vi "AFMss_control_trajTrack.vi"() -> ()   [LabVIEW 2017]
uses:
  controls/controlParams_tracktraj.ctl
  <vilib>/rvi/Emulation/niFpgaGetClockAttributes.vi
  <vilib>/rvi/Emulation/niFpgaSctlEmulationGetInTimedLoop.vi
  <vilib>/rvi/Emulation/niFpgaEmulationReportErrorSimple.vi
  <vilib>/rvi/eio/common/nirviEmuTemplateMethod_errors.vi
  <vilib>/rvi/Emulation/niFpgaCriticalErrorInLSC.vi
  <vilib>/rvi/DataTransferAndStorage/Container/Common/niFpgaContainerExecOnDevCompGetState.vi
  <vilib>/rvi/Emulation/niFpgaEmulationIsFPGAContextNoSignature.vi
  <vilib>/rvi/DataTransferAndStorage/Container/Common/niFpgaContainerGetUniqueNameForEmu.vi
  <vilib>/rvi/Memory/Memory_Emulation/niFpgaMemoryEmulationCacheClearOnFirstRun.vi
  <vilib>/rvi/Memory/Memory_Emulation/nirvimemoryEmulationManagerCache_MakeExclusive.vi
  <vilib>/rvi/Memory/Memory_Emulation/niFpgaMemoryEmulationValidateCache.vi
  <vilib>/rvi/Memory/Memory_Emulation/nirvimemoryEmulationManagerCache_InsertValue.vi
  <vilib>/Utility/error.llb/Clear Errors.vi
  <vilib>/rvi/Memory/Memory_Emulation/nirvimemoryEmulationManagerCache_ReleaseExclusive.vi
  <vilib>/rvi/Memory/Memory_Emulation/nirvimemoryEmulationManagerCache_GetValue.vi
  <vilib>/rvi/Memory/Memory_Emulation/nirvimemoryEmulationManagerCache_SetValue.vi
  <vilib>/rvi/Emulation/niFpgaProcessEmulError.vi
  <vilib>/rvi/interface/RandomDataEmulation/niFpgaRandomDataHandleErrors.vi
  <vilib>/eio/EIONode/EIONode.xnode
  <vilib>/rvi/DataTransferAndStorage/Container/XNode/niFpgaContainer.xnode
  <vilib>/rvi/DataTransferAndStorage/Register/Emulation/niFpgaRegisterEmulationRefIn.vi
  <vilib>/rvi/interface/RandomDataEmulation/nirviRandomDataFpgaReadWriteTemplate.vi
  <vilib>/rvi/FXPMathLib/FxpSub/XNode/nifxpmath_Sub.xnode
  <vilib>/rvi/FXPMathLib/sim/FxpSim.dll
panel:
  out "yk":sgl
  out "u_xk":sgl
  out "yuxk TO":bool
  out "YK TO":bool
  out "UK TO":bool
  in  "Cluster":T1={"umax"=3.0, "y_ref(k)"=0.0, "Ki"=0.0, "y(k) (from plant)"=0.0, "ND"=0, "NS"=0, "u_Kx_ref(k)"=0.0} {"u_Kx_ref(k)" format="%#_13g"; "Ki" format="%#_13g"; "y_ref(k)" format="%#_13g"; "umax" format="%#_13g"}
  out "Unstable Traj":bool
  out "Loop Done":bool
  in  "Settle Ticks":i16=1000
  in  "False  = cont run":bool=TRUE
  in  "Abort":bool=TRUE
  in  "iters":i16=1
  in  "ymax":sgl=4.0 format="%#_13g"
  in  "TsTicks":i16
  out "Loop Ticks (benchmark)":i16
  out "NS":i16=2
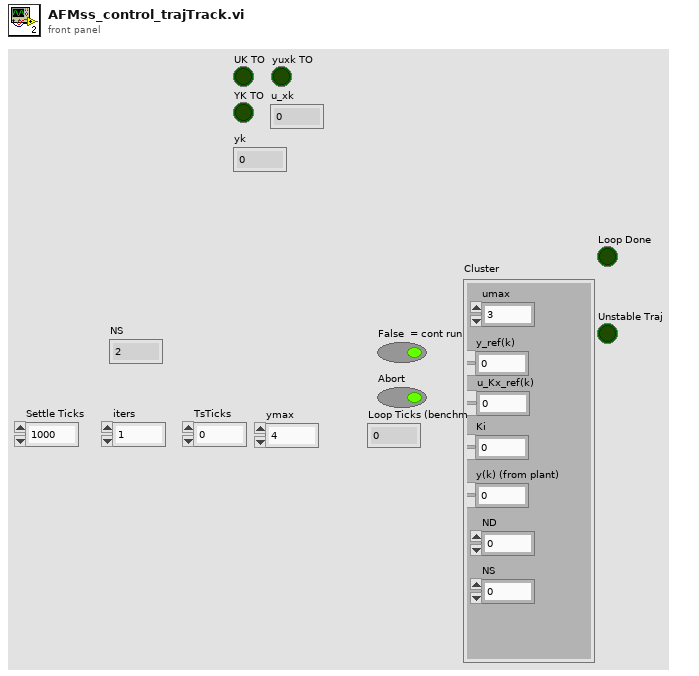
[diagram p1: front panel]
types:
  T1 = typedef "controlParams_tracktraj.ctl" = cluster{"umax":sgl, "y_ref(k)":sgl, "Ki":sgl, "y(k) (from plant)":sgl, "ND":i16, "NS":i16, "u_Kx_ref(k)":sgl}
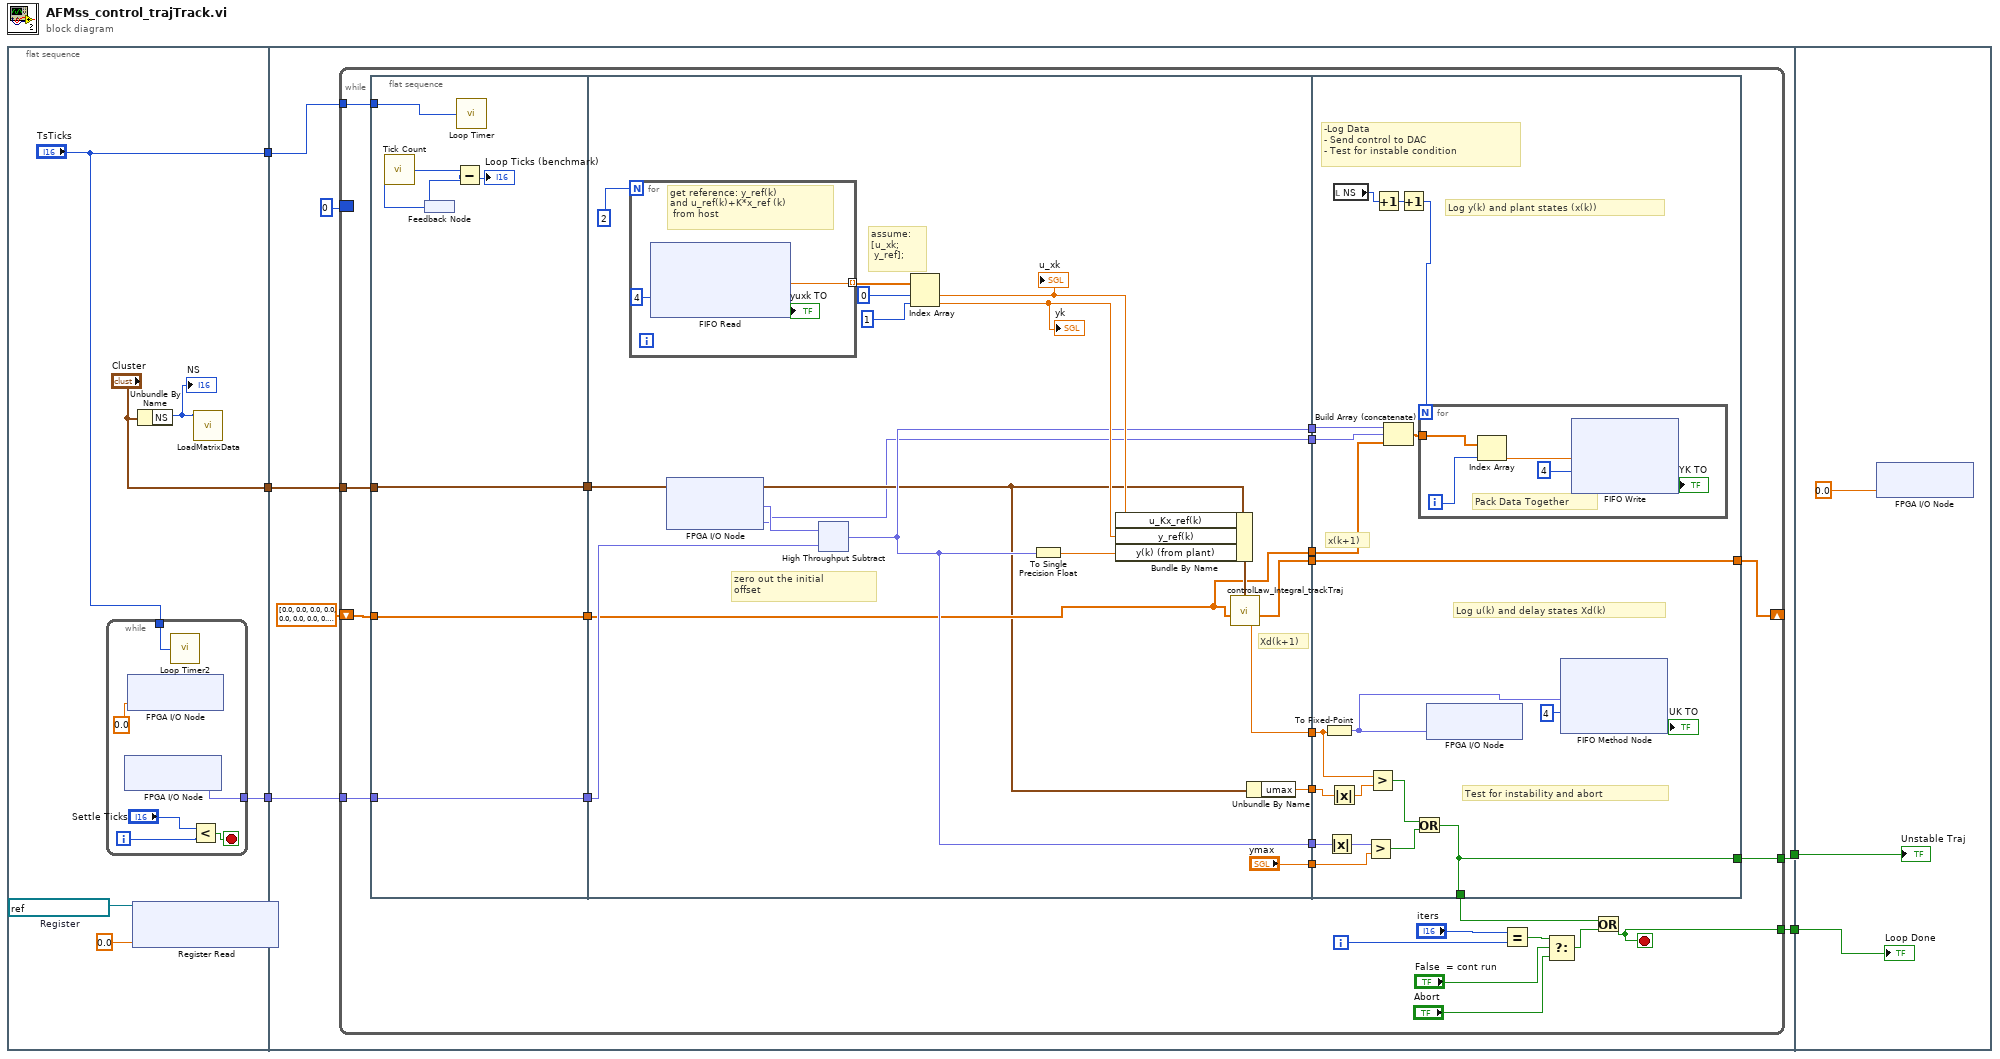
[diagram p0: block diagram]
diagram:
  n1 = flat-sequence {
    tunnel: ["TsTicks"] -> w5
    tunnel: [w11] -> w4
    tunnel: ["Cluster"] -> w2
    tunnel: w5 -> [w23]
    tunnel: w4 -> [w22]
    tunnel: [w20] -> w3
    tunnel: w2 -> [w19]
    tunnel: [w18] -> w1
    tunnel: w3 -> [w104]
    tunnel: w1 -> [w103]
    frame #0 {
      w9 = refnum<k21> "accumulator"  # Register
      # "Load Matrix Data"
      n2 = while {
        tunnel: [w17] -> w11
        tunnel: "TsTicks" -> [w16]
        i -> [w12]
        stop <- w14 stop-if-true
        n3 = xnode "FPGA I/O Node"() -> ("Mod2/AI0"=w17:fxp<+/-,24,5>)  [unwired: 1 in, 1 out]
        n4 = xnode "FPGA I/O Node"("Mod1/AO0"=sgl 0.0) -> ()  [unwired: 1 in, 1 out]
        n5 = call "Loop Timer2"("Count(Ticks)"=w16) -> ()  [unwired: 1 out]
        n6 = Less?(x="Settle Ticks", y=w12) -> (x < y?=w14:bool)
      }
      n7 = xnode ("Register Read")("Data"=sgl 0.0, "Register In"=w9) -> ()  [unwired: 1 out]
      n8 = Unbundle By Name("Cluster") -> ("NS"=w6:i16)
      "NS" <- w6
      n9 = call "LoadMatrixData.vi"("NS"=w6) -> ()  [unwired: 10 in, 1 out]
    }
    frame #1 {
      n10 = while {
        border: i16 0 -> [_]
        tunnel: w23 -> [w40]
        tunnel: w22 -> [w38]
        shift-right: [w30] -> _
        shift-left: sgl[] [0.0, 0.0, 0.0, 0.0, 0.0, 0.0, 0.0, 0.0, 0.0, 0.0, 0.0, 0.0, 0.0, 0.0, 0.0, 0.0, 0.0, 0.0, 0.0, 0.0, 0.0, 0.0, 0.0, 0.0, 0.0] ("x^(k+1) = Ax + Bu + Lye") -> [w36]
        tunnel: [w34] -> w20
        tunnel: w19 -> [w32]
        tunnel: [w31] -> w18
        i -> [w45]
        stop <- w34 stop-if-true
        n11 = flat-sequence {
          tunnel: w40 -> [w53]
          tunnel: w38 -> [w52]
          tunnel: [w52] -> w37
          tunnel: w36 -> [w51]
          tunnel: [w51] -> w35
          tunnel: [w50] -> w33
          tunnel: w32 -> [w50]
          tunnel: [w62] -> w49
          tunnel: [w64] -> w48
          tunnel: [w66] -> w39
          tunnel: w37 -> [w74]
          tunnel: w35 -> [w63]
          tunnel: w33 -> [w61]
          tunnel: [w63] -> w29
          tunnel: [w66] -> w28
          tunnel: [w60] -> w27
          tunnel: ["ymax"] -> w26
          tunnel: [w57] -> w25
          tunnel: w49 -> [w95]
          tunnel: w48 -> [w89]
          tunnel: [w83] -> w47
          tunnel: w39 -> [w81]
          tunnel: [w83] -> w31
          tunnel: [w95] -> w30
          tunnel: w29 -> [w94]
          tunnel: w28 -> [w93]
          tunnel: w27 -> [w88]
          tunnel: w26 -> [w86]
          tunnel: w25 -> [w82]
          frame #0 {
            n12 = call "Tick Count"() -> ("Tick Count(Ticks)"=w54:u32)
            n13 = feedback #1() -> (w55:u32)
            n14 = feedback-in #1(w54) -> ()
            n15 = Subtract(x=w54, y=w55) -> (x-y=→"Loop Ticks (benchmark)":u32)
            n16 = call "Loop Timer"("Count(Ticks)"=w53) -> ()  [unwired: 1 out]
          }
          frame #1 {
            # "assume:\n[u_xk;\n y_ref];"
            # "Xd(k+1)"
            # "zero out the initial \noffset"
            n17 = for {
              N: i16 2 -> [_]
              tunnel: [w76] -> w71 mode=indexing
              # "get reference: y_ref(k)\nand u_ref(k)+K*x_ref (k)\n from host"
              n18 = xnode ("FIFO Read")("Timeout"=i16 4) -> ("Element"=w76:sgl, "Timed Out?"=→"yuxk TO":bool)  [unwired: 1 in, 1 out]
            }
            n19 = xnode "FPGA I/O Node"() -> ("Mod2/AI0"=w58:fxp<+/-,24,5>, "Mod2/AI2"=w57:fxp<+/-,24,5>)  [unwired: 2 in, 2 out]
            n20 = xnode "High Throughput Subtract"("x"=w58, "y"=w74) -> ("x-y"=w66:fxp<+/-,40,6>)
            n21 = Index Array(array=w71, index #1=i16 0, index #2=i16 1) -> (element #1=w68:sgl, element #2=w67:sgl)
            "u_xk" <- w68
            "yk" <- w67
            n22 = To Single Precision Float(number=w66) -> (single precision float=w73:sgl)
            n23 = Bundle By Name(cluster=w61, "u_Kx_ref(k)"=w68, "y_ref(k)"=w67, "y(k) (from plant)"=w73) -> (w65:T1)
            n24 = call "controlLaw_Integral_trackTraj.vi"("Cluster"=w65, "x^(k)"=w63) -> ("x^(k+1) = Ax + Bu + Lye"=w62:sgl[], "u(k) (saturated)"=w64:sgl)  [unwired: 8 in]
            n25 = Unbundle By Name(w61) -> ("umax"=w60:sgl)
          }
          frame #2 {
            # "x(k+1)"
            # "Log u(k) and delay states Xd(k)"
            # "Log y(k) and plant states (x(k))"
            # "-Log Data\n- Send control to DAC\n- Test for instable condition"
            # "Test for instability and abort"
            n26 = To Fixed-Point(number=w89) -> (fixed-point=w92:fxp<+/-,32,6>)  [unwired: 1 in]
            n27 = Absolute Value(x=w93) -> (abs(x)=w97:fxp<+,40,6>)
            n28 = Absolute Value(x=w88) -> (abs(x)=w87:sgl)
            n29 = local read "NS"() -> (w78:i16)
            n30 = Greater?(x=w97, y=w86) -> (0:w84:bool)
            n31 = Greater?(x=w89, y=w87) -> (0:w85:bool)
            n32 = Increment(x=w78) -> (x+1=w80:i16)
            n33 = Build Array (concatenate)(w81, w82, w94) -> (w96:sgl[])
            n34 = Increment(x=w80) -> (x+1=w79:i16)
            n35 = Or(x=w85, y=w84) -> (x .or. y?=w83:bool)
            n36 = for {
              N: w79 -> [_]
              tunnel: w96 -> [w100]
              i -> [w101]
              # "Pack Data Together"
              n37 = Index Array(array=w100, index=w101) -> (element=w99:sgl)
              n38 = xnode ("FIFO Write")("Element"=w99, "Timeout"=i16 4) -> ("Timed Out?"=→"YK TO":bool)  [unwired: 1 in, 1 out]
            }
            n39 = xnode "FPGA I/O Node"("Mod1/AO0"=w92) -> ()  [unwired: 1 in, 1 out]
            n40 = xnode ("FIFO Method Node")("Element"=w92, "Timeout"=i16 4) -> ("Timed Out?"=→"UK TO":bool)  [unwired: 1 in, 1 out]
          }
        }
        n41 = Equal?(x="iters", y=w45) -> (x = y?=w43:bool)
        n42 = Select(t=w43, s="False  = cont run", f="Abort") -> (s? t:f=w44:bool)
        n43 = Or(x=w47, y=w44) -> (x .or. y?=w34:bool)
      }
    }
    frame #2 {
      n44 = xnode "FPGA I/O Node"("Mod1/AO0"=sgl 0.0) -> ()  [unwired: 1 in, 1 out]
      "Loop Done" <- w104
      "Unstable Traj" <- w103
    }
  }
